vi "Exit.vi"(8 "error in (no error)":errorcluster, 11 "Exit? (T)":bool=TRUE) -> (0 "error out":errorcluster)   [LabVIEW 2018, in "Error Handler.lvlib"]
doc: "This subVI enqueues the named action in to the communications queue along with the input data."
uses:
  Error Handler.lvlib
  Private Controls/Module Data.ctl
  Private Controls/Module Action.ctl
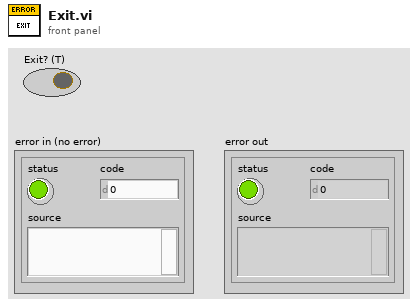
[diagram p1: front panel]
types:
  T1 = typedef "Error Handler.lvlib/Module Data.ctl" = cluster{"Data":variant, "Action":T2}
  T2 = typedef "Error Handler.lvlib/Module Action.ctl" = enum8{"Init", "Error", "Exit", "Module Error", "Controller Error", "UI1 Error", "UI2 Error", "UI3 Error", "File IO Error", "cRIO Error", "Calibration Error"}
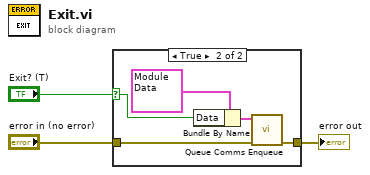
[diagram p0: block diagram]
diagram:
  n1 = case shown="True" "Exit? (T)" {
    selector: "Exit? (T)" -> [_ w9]
    tunnel: "error in (no error)" -> [w4 w7]
    tunnel: [w4 w6] -> w2
    frame False {
    }
    frame True {
      n2 = Bundle By Name(cluster=T1 {"Data"=variant, "Action"=enum."Exit"} ("element"), "Data"=w9) -> (w5:T1)
      n3 = call "Queue Comms Enqueue.vi"("error in (no error)"=w7, "element"=w5) -> ("error out"=w6:errorcluster)  [unwired: 9 in]
    }
  }
  "error out" <- w2
